vi "SwissSPAD Live_Settings Storage.vi"(6 "Set/Get(F)":bool, 7 "Settings List":T15=enum."FPGA:Bottom Bitfile Path", 8 "Error In":errorcluster, 11 "Variant Data in":variant) -> (0 "Error Out":errorcluster, 3 "Variant Data out":variant)   [LabVIEW 2021]
uses:
  SwissSPAD Live_Settings List.ctl
  SwissSPAD Live_SS2 DAQ Parameters 3.ctl
  SwissSPAD Live_SS2 Gate Definition.ctl
  SwissSPAD Live_File Information.ctl
  SwissSPAD Live_SS2 Gate Configuration.ctl
  SwissSPAD Live_Image ROI Information.ctl
  Phasor/Image Binning Options.ctl
  SwissSPAD Live_SS3 DAQ Parameters.ctl
  SwissSPAD Live_SS3 Gate Definition.ctl
  SS3 Gate Width Definition Mode.ctl
  SwissSPAD Live_SS3 Displayed Image v2.ctl
  SwissSPAD Live_SSx PCB Version.ctl
  SwissSPAD Live_Image Display Options.ctl
  SwissSPAD Live_FPGA Data to Display.ctl
  281105eb-bd69-41f7-a288-d5f8cce70846.vi
panel:
  in  "Tab Control":T1(tab)
  in  "Top Half":bool
  in  "Top FPGA Serial Number":string
  in  "Top Bitstream Version":string
  in  "Top Bitfile Path":path
  in  "Bottom Half":bool
  in  "Detector PCB Version":T2
  in  "Bottom FPGA Serial Number":string
  in  "Bottom Bitstream Version":string
  in  "Bottom BitFile Path":path
  in  "Auto Reset FPGA":bool
  in  "Microlens":bool
  in  "SS3 DAQ Parameters":T3={"10 bits"=FALSE, "# Exposure Sequences"=0, "# 1-bit Frame per Gate"=255, "Gate Shift"=0, "# Gate Pairs per Set"=0, "# Sets"=1, "Laser Period"=0.0, "Sync Period"=0.0, "Gate Offset"=0, "Auto-adjust Gate Offset"=FALSE, "Gate Definition"={"gs_psincdec_0"=0, "gs_psincdec_1"=0, "gs_no_shift_adj_1"=0, "gate_adj_2"=0}, "Gate Width (ns)"=0.0, "Reversed Shift"=FALSE, "Intensity Mode"=FALSE, "Gate Definition Mode"=enum."Item 0"} {"Gate Width (ns)" min=0.0 max=100.0 format="%#_5g"; "# Sets" min=1}
  in  "Buffer Size (# 8-bit Gates)":u32=1 min=1
  in  "SS2 DAQ Parameters":T6 {"Sync Period" min=0.0 max=4.294967295; "Laser Period" min=0.0 max=4.294967295}
  in  "Gate Configuration Definitions":T8[](array[typedef])
  in  "FPGA Data to Display":T9
  in  "Use Histogram Cursors":bool
  in  "Image Display Options":T10 {"Percentile" min=0 max=100}
  in  "Image Binning Options":T11={"Use Image Binning"=FALSE, "X Bin"=1, "Y Bin"=1} {"Y Bin" min=1; "X Bin" min=1}
  in  "Image ROI Information":T12
  in  "SS3 Displayed Image":T13
  in  "Save Sum of All Gates Preview":bool
  in  "SS3 Gate Slip Correction":bool
  in  "Delay between Datasets":dbl[unit]
  in  "Scrambled File Flag":bool
  in  "# Datasets in Series":i32=1 min=1
  in  "File Information":T14={"File Folder"=path "", "File Name"="", "File Index"=0, "Author"="", "Sample"="", "Compression"=FALSE, "Compression Level"=9} {"Compression Level" max=9}
  in  "SS3 Hot Pixel Mismatch Detection":bool
  in  "Histogram Bin Size":i32=256 min=1 step=1
  in  "Verbose Saving":bool
  in  "Verbose Settings":bool
  in  "Use Image Display Options":bool
  in  "# Histogram Bins":i32=1 min=1 step=1
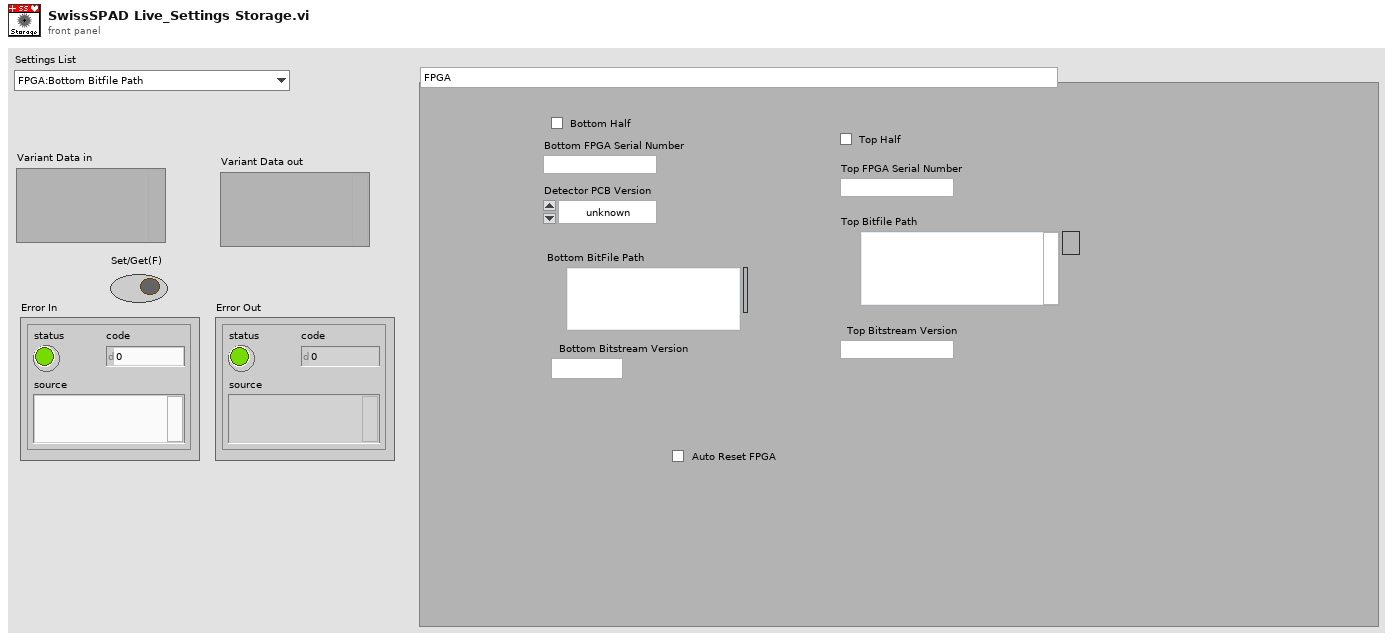
[diagram p1: front panel]
types:
  T1 = enum32{"FPGA", "Acquisition Parameters", "Image Parameters", "File Information", "UI Settings"}
  T2 = typedef "SwissSPAD Live_SSx PCB Version.ctl" = enum16{"unknown", "SS2 PCB1", "SS2 PCB2", "SS3 PCB1"}
  T3 = typedef "SwissSPAD Live_SS3 DAQ Parameters.ctl" = cluster{"10 bits":bool, "# Exposure Sequences":u32, "# 1-bit Frame per Gate":u32, "Gate Shift":u32, "# Gate Pairs per Set":u32, "# Sets":u32, "Laser Period":dbl[unit], "Sync Period":dbl[unit], "Gate Offset":u32, "Auto-adjust Gate Offset":bool, "Gate Definition":T4, "Gate Width (ns)":dbl, "Reversed Shift":bool, "Intensity Mode":bool, "Gate Definition Mode":T5}
  T4 = typedef "SwissSPAD Live_SS3 Gate Definition.ctl" = cluster{"gs_psincdec_0":u32, "gs_psincdec_1":u32, "gs_no_shift_adj_1":u32, "gate_adj_2":u32}
  T5 = typedef "SS3 Gate Width Definition Mode.ctl" = enum32{"Item 0", "Item 1"}
  T6 = typedef "SwissSPAD Live_SS2 DAQ Parameters 3.ctl" = cluster{"10 bits":bool, "# Exposure Sequences":u32, "# 1-bit Frame per Gate":u32, "Gate Shift":u32, "# Gates per Set":u32, "# Sets":u32, "Laser Period":dbl[unit], "Sync Period":dbl[unit], "Gate Offset":u32, "Auto-adjust Gate Offset":bool, "Gate Definition":T7, "Reversed Shift":bool}
  T7 = typedef "SwissSPAD Live_SS2 Gate Definition.ctl" = cluster{"gs_psincdec_0":u32, "gs_psincdec_1":u32, "gs_psincdec_2":u32, "gs_psincdec_3":u32, "gs_no_shift_adj_1":u32, "gs_no_shift_adj_2":u32, "gs_no_shift_adj_3":u32}
  T8 = typedef "SwissSPAD Live_SS2 Gate Configuration.ctl" = cluster{"Gate Configuration":string, "Gate Offset":u32, "Gate Definition":T7}
  T9 = typedef "SwissSPAD Live_FPGA Data to Display.ctl" = enum16{"Bottom FPGA", "Top FPGA", "Both"}
  T10 = typedef "SwissSPAD Live_Image Display Options.ctl" = cluster{"Remove Screamers":bool, "Delta":sgl, "Equalize Histogram":bool, "Percentile":sgl, "Hot Pixel Mask Image":path, "Use Hot Pixel Mask":bool}
  T11 = typedef "Image Binning Options.ctl" = cluster{"Use Image Binning":bool, "X Bin":i32, "Y Bin":i32}
  T12 = typedef "SwissSPAD Live_Image ROI Information.ctl" = cluster{"Save ROI Only":bool, "Left":u16, "Top":u16, "Right":u16, "Bottom":u16, "Use Current ROI":bool}
  T13 = typedef "SwissSPAD Live_SS3 Displayed Image v2.ctl" = enum16{"G2 Gate", "INT Gate", "INT - G2"}
  T14 = typedef "SwissSPAD Live_File Information.ctl" = cluster{"File Folder":path, "File Name":string, "File Index":u32, "Author":string, "Sample":string, "Compression":bool, "Compression Level":u8}
  T15 = typedef "SwissSPAD Live_Settings List.ctl" = enum16{"FPGA:Bottom Half", "FPGA:Top Half", "FPGA:Bottom Bitfile Path", "FPGA:Top Bitfile Path", "FPGA:Bottom Bitstream Version", "FPGA:Top Bitstream Version", "FPGA:Auto Reset FPGA", "FPGA:Bottom FPGA Serial Number", "FPGA:Top FPGA Serial Number", "FPGA:Detector PCB Version", "Acquisition Parameters:Microlens", "Acquisition Parameters:SS2 DAQ Parameters", "Acquisition Parameters:Gate Configuration Array", "Acquisition Parameters:SS3 DAQ Parameters", "Acquisition Parameters:Buffer Size (# 8-bit Gates)", "File Information:File Information", "File Information:# Datasets in Series", "File Information:Scrambled File Flag", "File Information:SS3 Gate Slip Correction", "File Information:SS3 Hot Pixel Mismatch Detection", "File Information:Delay between Datasets", "File Information:Save Sum of All Gates Preview", "Image Parameters:Image ROI Information", "Image Parameters:Image Binning Options", "Image Parameters:SS3 Displayed Image", "Image Parameters:Image Display Options", "Image Parameters:Use Histogram Cursors", "Image Parameter:FPGA Data to Display", "UI Settings:Histogram Bins Number", "UI Settings:Histogram Bin Size", "UI Settings:Use Image Display Options", "UI Settings:Verbose Settings", "UI Settings:Verbose Saving"}
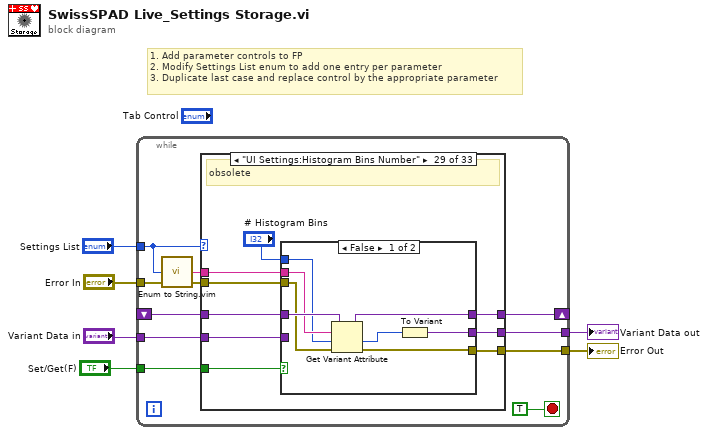
[diagram p0: block diagram]
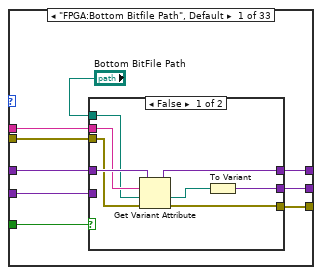
[diagram p2: hidden frame]
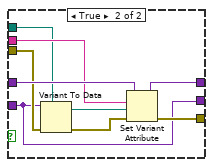
[diagram p3: hidden frame]
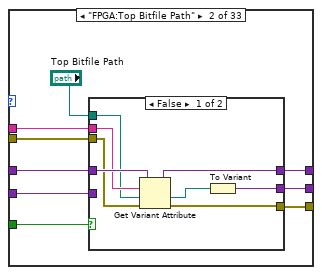
[diagram p4: hidden frame]
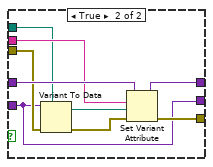
[diagram p5: hidden frame]
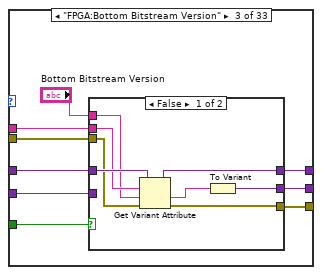
[diagram p6: hidden frame]
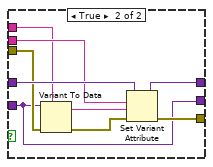
[diagram p7: hidden frame]
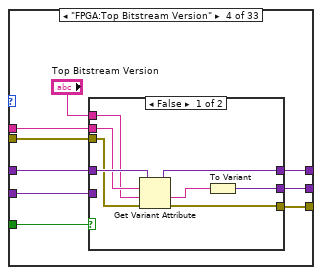
[diagram p8: hidden frame]
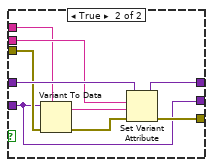
[diagram p9: hidden frame]
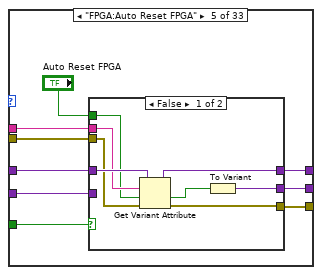
[diagram p10: hidden frame]
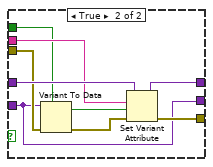
[diagram p11: hidden frame]
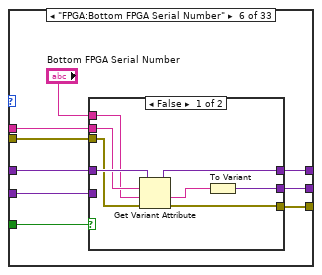
[diagram p12: hidden frame]
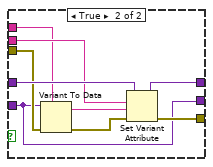
[diagram p13: hidden frame]
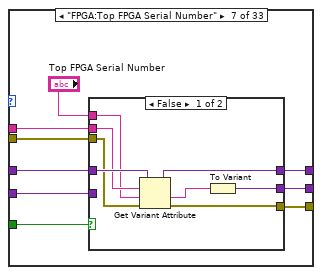
[diagram p14: hidden frame]
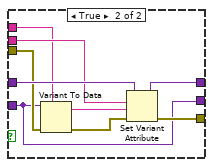
[diagram p15: hidden frame]
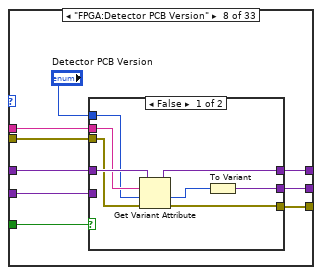
[diagram p16: hidden frame]
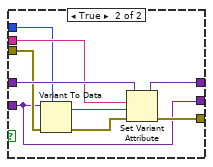
[diagram p17: hidden frame]
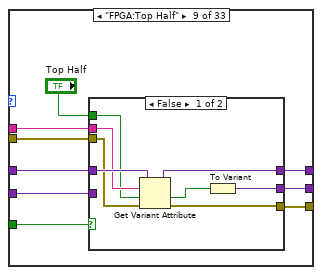
[diagram p18: hidden frame]
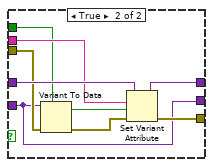
[diagram p19: hidden frame]
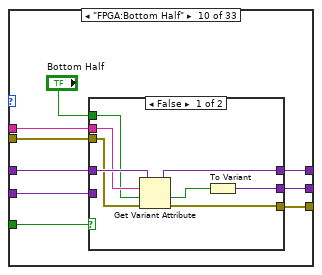
[diagram p20: hidden frame]
diagram:
  # "1. Add parameter controls to FP\n2. Modify Settings List enum to add one entry per parameter\n3. Duplicate last case and replace control by the appropriate parameter"
  n1 = while {
    tunnel: "Settings List" -> [w9]
    tunnel: "Error In" -> [w7]
    tunnel: "Set/Get(F)" -> [w15]
    shift-right: [w13] -> _
    shift-left: _ -> [w14]
    tunnel: "Variant Data in" -> [w12]
    tunnel: [w11] -> w2
    tunnel: [w10] -> w1
    stop <- TRUE stop-if-true
    n2 = call "Enum to String.vim"("Enum"=w9) -> ("String"=w8:string)
    n3 = case shown="\"UI Settings:Histogram Bins Number\"" w9 {
      tunnel: w15 -> [w25 w51 w77 w103 w129 w155 w181 w207 w233 w259 w285 w311 w337 w363 w389 w415 w441 w467 w493 w519 w545 w571 w597 w623 w649 w675 w701 w727 w753 w779 w805 w831 w857]
      tunnel: w14 -> [w24 w50 w76 w102 w128 w154 w180 w206 w232 w258 w284 w310 w336 w362 w388 w414 w440 w466 w492 w518 w544 w570 w596 w622 w648 w674 w700 w726 w752 w778 w804 w830 w856]
      tunnel: w8 -> [w23 w49 w75 w101 w127 w153 w179 w205 w231 w257 w283 w309 w335 w361 w387 w413 w439 w465 w491 w517 w543 w569 w595 w621 w647 w673 w699 w725 w751 w777 w803 w829 w855]
      tunnel: [w22 w48 w74 w100 w126 w152 w178 w204 w230 w256 w282 w308 w334 w360 w386 w412 w438 w464 w490 w516 w542 w568 w594 w620 w646 w672 w698 w724 w750 w776 w802 w828 w854] -> w13
      tunnel: w7 -> [w21 w47 w73 w99 w125 w151 w177 w203 w229 w255 w281 w307 w333 w359 w385 w411 w437 w463 w489 w515 w541 w567 w593 w619 w645 w671 w697 w723 w749 w775 w801 w827 w853]
      tunnel: w12 -> [w20 w46 w72 w98 w124 w150 w176 w202 w228 w254 w280 w306 w332 w358 w384 w410 w436 w462 w488 w514 w540 w566 w592 w618 w644 w670 w696 w722 w748 w774 w800 w826 w852]
      tunnel: [w19 w45 w71 w97 w123 w149 w175 w201 w227 w253 w279 w305 w331 w357 w383 w409 w435 w461 w487 w513 w539 w565 w591 w617 w643 w669 w695 w721 w747 w773 w799 w825 w851] -> w11
      tunnel: [w18 w44 w70 w96 w122 w148 w174 w200 w226 w252 w278 w304 w330 w356 w382 w408 w434 w460 w486 w512 w538 w564 w590 w616 w642 w668 w694 w720 w746 w772 w798 w824 w850] -> w10
      frame "FPGA:Bottom Bitfile Path", Default {
        n4 = case shown="False" w25 {
          tunnel: w24 -> [w33 w42]
          tunnel: w23 -> [w32 w41]
          tunnel: [w30 w40] -> w22
          tunnel: "Bottom BitFile Path" -> [w27 w39]
          tunnel: w21 -> [w31 w38]
          tunnel: w20 -> [_ w34]
          tunnel: [w29 w35] -> w19
          tunnel: [w26 w34] -> w18
          frame False {
            n5 = Get Variant Attribute(Variant=w33, name=w32, default value (empty Variant)=w27, error in=w31) -> (duplicate Variant=w30:variant, value=w28:path, error out=w29:errorcluster)  [unwired: 1 out]
            n6 = To Variant(anything=w28) -> (Variant=w26:variant)
          }
          frame True {
            n7 = Variant To Data(error in=w38, type=w39, Variant=w34) -> (data=w37:path, error out=w36:errorcluster)
            n8 = Set Variant Attribute(Variant=w42, name=w41, value=w37, error in=w36) -> (Variant out=w40:variant, error out=w35:errorcluster)  [unwired: 1 out]
          }
        }
      }
      frame "FPGA:Top Bitfile Path" {
        n9 = case shown="False" w51 {
          tunnel: w50 -> [w59 w68]
          tunnel: w49 -> [w58 w67]
          tunnel: [w56 w66] -> w48
          tunnel: "Top Bitfile Path" -> [w53 w65]
          tunnel: w47 -> [w57 w64]
          tunnel: w46 -> [_ w60]
          tunnel: [w55 w61] -> w45
          tunnel: [w52 w60] -> w44
          frame False {
            n10 = Get Variant Attribute(Variant=w59, name=w58, default value (empty Variant)=w53, error in=w57) -> (duplicate Variant=w56:variant, value=w54:path, error out=w55:errorcluster)  [unwired: 1 out]
            n11 = To Variant(anything=w54) -> (Variant=w52:variant)
          }
          frame True {
            n12 = Variant To Data(error in=w64, type=w65, Variant=w60) -> (data=w63:path, error out=w62:errorcluster)
            n13 = Set Variant Attribute(Variant=w68, name=w67, value=w63, error in=w62) -> (Variant out=w66:variant, error out=w61:errorcluster)  [unwired: 1 out]
          }
        }
      }
      frame "FPGA:Bottom Bitstream Version" {
        n14 = case shown="False" w77 {
          tunnel: w76 -> [w85 w94]
          tunnel: w75 -> [w84 w93]
          tunnel: [w82 w92] -> w74
          tunnel: "Bottom Bitstream Version" -> [w79 w91]
          tunnel: w73 -> [w83 w90]
          tunnel: w72 -> [_ w86]
          tunnel: [w81 w87] -> w71
          tunnel: [w78 w86] -> w70
          frame False {
            n15 = Get Variant Attribute(Variant=w85, name=w84, default value (empty Variant)=w79, error in=w83) -> (duplicate Variant=w82:variant, value=w80:string, error out=w81:errorcluster)  [unwired: 1 out]
            n16 = To Variant(anything=w80) -> (Variant=w78:variant)
          }
          frame True {
            n17 = Variant To Data(error in=w90, type=w91, Variant=w86) -> (data=w89:string, error out=w88:errorcluster)
            n18 = Set Variant Attribute(Variant=w94, name=w93, value=w89, error in=w88) -> (Variant out=w92:variant, error out=w87:errorcluster)  [unwired: 1 out]
          }
        }
      }
      frame "FPGA:Top Bitstream Version" {
        n19 = case shown="False" w103 {
          tunnel: w102 -> [w111 w120]
          tunnel: w101 -> [w110 w119]
          tunnel: [w108 w118] -> w100
          tunnel: "Top Bitstream Version" -> [w105 w117]
          tunnel: w99 -> [w109 w116]
          tunnel: w98 -> [_ w112]
          tunnel: [w107 w113] -> w97
          tunnel: [w104 w112] -> w96
          frame False {
            n20 = Get Variant Attribute(Variant=w111, name=w110, default value (empty Variant)=w105, error in=w109) -> (duplicate Variant=w108:variant, value=w106:string, error out=w107:errorcluster)  [unwired: 1 out]
            n21 = To Variant(anything=w106) -> (Variant=w104:variant)
          }
          frame True {
            n22 = Variant To Data(error in=w116, type=w117, Variant=w112) -> (data=w115:string, error out=w114:errorcluster)
            n23 = Set Variant Attribute(Variant=w120, name=w119, value=w115, error in=w114) -> (Variant out=w118:variant, error out=w113:errorcluster)  [unwired: 1 out]
          }
        }
      }
      frame "FPGA:Auto Reset FPGA" {
        n24 = case shown="False" w129 {
          tunnel: w128 -> [w137 w146]
          tunnel: w127 -> [w136 w145]
          tunnel: [w134 w144] -> w126
          tunnel: "Auto Reset FPGA" -> [w131 w143]
          tunnel: w125 -> [w135 w142]
          tunnel: w124 -> [_ w138]
          tunnel: [w133 w139] -> w123
          tunnel: [w130 w138] -> w122
          frame False {
            n25 = Get Variant Attribute(Variant=w137, name=w136, default value (empty Variant)=w131, error in=w135) -> (duplicate Variant=w134:variant, value=w132:bool, error out=w133:errorcluster)  [unwired: 1 out]
            n26 = To Variant(anything=w132) -> (Variant=w130:variant)
          }
          frame True {
            n27 = Variant To Data(error in=w142, type=w143, Variant=w138) -> (data=w141:bool, error out=w140:errorcluster)
            n28 = Set Variant Attribute(Variant=w146, name=w145, value=w141, error in=w140) -> (Variant out=w144:variant, error out=w139:errorcluster)  [unwired: 1 out]
          }
        }
      }
      frame "FPGA:Bottom FPGA Serial Number" {
        n29 = case shown="False" w155 {
          tunnel: w154 -> [w163 w172]
          tunnel: w153 -> [w162 w171]
          tunnel: [w160 w170] -> w152
          tunnel: "Bottom FPGA Serial Number" -> [w157 w169]
          tunnel: w151 -> [w161 w168]
          tunnel: w150 -> [_ w164]
          tunnel: [w159 w165] -> w149
          tunnel: [w156 w164] -> w148
          frame False {
            n30 = Get Variant Attribute(Variant=w163, name=w162, default value (empty Variant)=w157, error in=w161) -> (duplicate Variant=w160:variant, value=w158:string, error out=w159:errorcluster)  [unwired: 1 out]
            n31 = To Variant(anything=w158) -> (Variant=w156:variant)
          }
          frame True {
            n32 = Variant To Data(error in=w168, type=w169, Variant=w164) -> (data=w167:string, error out=w166:errorcluster)
            n33 = Set Variant Attribute(Variant=w172, name=w171, value=w167, error in=w166) -> (Variant out=w170:variant, error out=w165:errorcluster)  [unwired: 1 out]
          }
        }
      }
      frame "FPGA:Top FPGA Serial Number" {
        n34 = case shown="False" w181 {
          tunnel: w180 -> [w189 w198]
          tunnel: w179 -> [w188 w197]
          tunnel: [w186 w196] -> w178
          tunnel: "Top FPGA Serial Number" -> [w183 w195]
          tunnel: w177 -> [w187 w194]
          tunnel: w176 -> [_ w190]
          tunnel: [w185 w191] -> w175
          tunnel: [w182 w190] -> w174
          frame False {
            n35 = Get Variant Attribute(Variant=w189, name=w188, default value (empty Variant)=w183, error in=w187) -> (duplicate Variant=w186:variant, value=w184:string, error out=w185:errorcluster)  [unwired: 1 out]
            n36 = To Variant(anything=w184) -> (Variant=w182:variant)
          }
          frame True {
            n37 = Variant To Data(error in=w194, type=w195, Variant=w190) -> (data=w193:string, error out=w192:errorcluster)
            n38 = Set Variant Attribute(Variant=w198, name=w197, value=w193, error in=w192) -> (Variant out=w196:variant, error out=w191:errorcluster)  [unwired: 1 out]
          }
        }
      }
      frame "FPGA:Detector PCB Version" {
        n39 = case shown="False" w207 {
          tunnel: w206 -> [w215 w224]
          tunnel: w205 -> [w214 w223]
          tunnel: [w212 w222] -> w204
          tunnel: "Detector PCB Version" -> [w209 w221]
          tunnel: w203 -> [w213 w220]
          tunnel: w202 -> [_ w216]
          tunnel: [w211 w217] -> w201
          tunnel: [w208 w216] -> w200
          frame False {
            n40 = Get Variant Attribute(Variant=w215, name=w214, default value (empty Variant)=w209, error in=w213) -> (duplicate Variant=w212:variant, value=w210:T2, error out=w211:errorcluster)  [unwired: 1 out]
            n41 = To Variant(anything=w210) -> (Variant=w208:variant)
          }
          frame True {
            n42 = Variant To Data(error in=w220, type=w221, Variant=w216) -> (data=w219:T2, error out=w218:errorcluster)
            n43 = Set Variant Attribute(Variant=w224, name=w223, value=w219, error in=w218) -> (Variant out=w222:variant, error out=w217:errorcluster)  [unwired: 1 out]
          }
        }
      }
      frame "FPGA:Top Half" {
        n44 = case shown="False" w233 {
          tunnel: w232 -> [w241 w250]
          tunnel: w231 -> [w240 w249]
          tunnel: [w238 w248] -> w230
          tunnel: "Top Half" -> [w235 w247]
          tunnel: w229 -> [w239 w246]
          tunnel: w228 -> [_ w242]
          tunnel: [w237 w243] -> w227
          tunnel: [w234 w242] -> w226
          frame False {
            n45 = Get Variant Attribute(Variant=w241, name=w240, default value (empty Variant)=w235, error in=w239) -> (duplicate Variant=w238:variant, value=w236:bool, error out=w237:errorcluster)  [unwired: 1 out]
            n46 = To Variant(anything=w236) -> (Variant=w234:variant)
          }
          frame True {
            n47 = Variant To Data(error in=w246, type=w247, Variant=w242) -> (data=w245:bool, error out=w244:errorcluster)
            n48 = Set Variant Attribute(Variant=w250, name=w249, value=w245, error in=w244) -> (Variant out=w248:variant, error out=w243:errorcluster)  [unwired: 1 out]
          }
        }
      }
      frame "FPGA:Bottom Half" {
        n49 = case shown="False" w259 {
          tunnel: w258 -> [w267 w276]
          tunnel: w257 -> [w266 w275]
          tunnel: [w264 w274] -> w256
          tunnel: "Bottom Half" -> [w261 w273]
          tunnel: w255 -> [w265 w272]
          tunnel: w254 -> [_ w268]
          tunnel: [w263 w269] -> w253
          tunnel: [w260 w268] -> w252
          frame False {
            n50 = Get Variant Attribute(Variant=w267, name=w266, default value (empty Variant)=w261, error in=w265) -> (duplicate Variant=w264:variant, value=w262:bool, error out=w263:errorcluster)  [unwired: 1 out]
            n51 = To Variant(anything=w262) -> (Variant=w260:variant)
          }
          frame True {
            n52 = Variant To Data(error in=w272, type=w273, Variant=w268) -> (data=w271:bool, error out=w270:errorcluster)
            n53 = Set Variant Attribute(Variant=w276, name=w275, value=w271, error in=w270) -> (Variant out=w274:variant, error out=w269:errorcluster)  [unwired: 1 out]
          }
        }
      }
      frame "Acquisition Parameters:Microlens" {
        n54 = case shown="False" w285 {
          tunnel: w284 -> [w293 w302]
          tunnel: w283 -> [w292 w301]
          tunnel: [w290 w300] -> w282
          tunnel: "Microlens" -> [w287 w299]
          tunnel: w281 -> [w291 w298]
          tunnel: w280 -> [_ w294]
          tunnel: [w289 w295] -> w279
          tunnel: [w286 w294] -> w278
          frame False {
            n55 = Get Variant Attribute(Variant=w293, name=w292, default value (empty Variant)=w287, error in=w291) -> (duplicate Variant=w290:variant, value=w288:bool, error out=w289:errorcluster)  [unwired: 1 out]
            n56 = To Variant(anything=w288) -> (Variant=w286:variant)
          }
          frame True {
            n57 = Variant To Data(error in=w298, type=w299, Variant=w294) -> (data=w297:bool, error out=w296:errorcluster)
            n58 = Set Variant Attribute(Variant=w302, name=w301, value=w297, error in=w296) -> (Variant out=w300:variant, error out=w295:errorcluster)  [unwired: 1 out]
          }
        }
      }
      frame "Acquisition Parameters:SS2 DAQ Parameters" {
        n59 = case shown="False" w311 {
          tunnel: w310 -> [w319 w328]
          tunnel: w309 -> [w318 w327]
          tunnel: [w316 w326] -> w308
          tunnel: "SS2 DAQ Parameters" -> [w313 w325]
          tunnel: w307 -> [w317 w324]
          tunnel: w306 -> [_ w320]
          tunnel: [w315 w321] -> w305
          tunnel: [w312 w320] -> w304
          frame False {
            n60 = Get Variant Attribute(Variant=w319, name=w318, default value (empty Variant)=w313, error in=w317) -> (duplicate Variant=w316:variant, value=w314:T6, error out=w315:errorcluster)  [unwired: 1 out]
            n61 = To Variant(anything=w314) -> (Variant=w312:variant)
          }
          frame True {
            n62 = Variant To Data(error in=w324, type=w325, Variant=w320) -> (data=w323:T6, error out=w322:errorcluster)
            n63 = Set Variant Attribute(Variant=w328, name=w327, value=w323, error in=w322) -> (Variant out=w326:variant, error out=w321:errorcluster)  [unwired: 1 out]
          }
        }
      }
      frame "Acquisition Parameters:SS3 DAQ Parameters" {
        n64 = case shown="False" w337 {
          tunnel: w336 -> [w345 w354]
          tunnel: w335 -> [w344 w353]
          tunnel: [w342 w352] -> w334
          tunnel: "SS3 DAQ Parameters" -> [w339 w351]
          tunnel: w333 -> [w343 w350]
          tunnel: w332 -> [_ w346]
          tunnel: [w341 w347] -> w331
          tunnel: [w338 w346] -> w330
          frame False {
            n65 = Get Variant Attribute(Variant=w345, name=w344, default value (empty Variant)=w339, error in=w343) -> (duplicate Variant=w342:variant, value=w340:T3, error out=w341:errorcluster)  [unwired: 1 out]
            n66 = To Variant(anything=w340) -> (Variant=w338:variant)
          }
          frame True {
            n67 = Variant To Data(error in=w350, type=w351, Variant=w346) -> (data=w349:T3, error out=w348:errorcluster)
            n68 = Set Variant Attribute(Variant=w354, name=w353, value=w349, error in=w348) -> (Variant out=w352:variant, error out=w347:errorcluster)  [unwired: 1 out]
          }
        }
      }
      frame "Acquisition Parameters:Gate Configuration Array" {
        n69 = case shown="False" w363 {
          tunnel: w362 -> [w371 w380]
          tunnel: w361 -> [w370 w379]
          tunnel: [w368 w378] -> w360
          tunnel: "Gate Configuration Definitions" -> [w365 w377]
          tunnel: w359 -> [w369 w376]
          tunnel: w358 -> [_ w372]
          tunnel: [w367 w373] -> w357
          tunnel: [w364 w372] -> w356
          frame False {
            n70 = Get Variant Attribute(Variant=w371, name=w370, default value (empty Variant)=w365, error in=w369) -> (duplicate Variant=w368:variant, value=w366:T8[], error out=w367:errorcluster)  [unwired: 1 out]
            n71 = To Variant(anything=w366) -> (Variant=w364:variant)
          }
          frame True {
            n72 = Variant To Data(error in=w376, type=w377, Variant=w372) -> (data=w375:T8[], error out=w374:errorcluster)
            n73 = Set Variant Attribute(Variant=w380, name=w379, value=w375, error in=w374) -> (Variant out=w378:variant, error out=w373:errorcluster)  [unwired: 1 out]
          }
        }
      }
      frame "Acquisition Parameters:Buffer Size (# 8-bit Gates)" {
        n74 = case shown="False" w389 {
          tunnel: w388 -> [w397 w406]
          tunnel: w387 -> [w396 w405]
          tunnel: [w394 w404] -> w386
          tunnel: "Buffer Size (# 8-bit Gates)" -> [w391 w403]
          tunnel: w385 -> [w395 w402]
          tunnel: w384 -> [_ w398]
          tunnel: [w393 w399] -> w383
          tunnel: [w390 w398] -> w382
          frame False {
            n75 = Get Variant Attribute(Variant=w397, name=w396, default value (empty Variant)=w391, error in=w395) -> (duplicate Variant=w394:variant, value=w392:u32, error out=w393:errorcluster)  [unwired: 1 out]
            n76 = To Variant(anything=w392) -> (Variant=w390:variant)
          }
          frame True {
            n77 = Variant To Data(error in=w402, type=w403, Variant=w398) -> (data=w401:u32, error out=w400:errorcluster)
            n78 = Set Variant Attribute(Variant=w406, name=w405, value=w401, error in=w400) -> (Variant out=w404:variant, error out=w399:errorcluster)  [unwired: 1 out]
          }
        }
      }
      frame "File Information:File Information" {
        n79 = case shown="False" w415 {
          tunnel: w414 -> [w423 w432]
          tunnel: w413 -> [w422 w431]
          tunnel: [w420 w430] -> w412
          tunnel: "File Information" -> [w417 w429]
          tunnel: w411 -> [w421 w428]
          tunnel: w410 -> [_ w424]
          tunnel: [w419 w425] -> w409
          tunnel: [w416 w424] -> w408
          frame False {
            n80 = Get Variant Attribute(Variant=w423, name=w422, default value (empty Variant)=w417, error in=w421) -> (duplicate Variant=w420:variant, value=w418:T14, error out=w419:errorcluster)  [unwired: 1 out]
            n81 = To Variant(anything=w418) -> (Variant=w416:variant)
          }
          frame True {
            n82 = Variant To Data(error in=w428, type=w429, Variant=w424) -> (data=w427:T14, error out=w426:errorcluster)
            n83 = Set Variant Attribute(Variant=w432, name=w431, value=w427, error in=w426) -> (Variant out=w430:variant, error out=w425:errorcluster)  [unwired: 1 out]
          }
        }
      }
      frame "File Information:# Datasets in Series" {
        n84 = case shown="False" w441 {
          tunnel: w440 -> [w449 w458]
          tunnel: w439 -> [w448 w457]
          tunnel: [w446 w456] -> w438
          tunnel: "# Datasets in Series" -> [w443 w455]
          tunnel: w437 -> [w447 w454]
          tunnel: w436 -> [_ w450]
          tunnel: [w445 w451] -> w435
          tunnel: [w442 w450] -> w434
          frame False {
            n85 = Get Variant Attribute(Variant=w449, name=w448, default value (empty Variant)=w443, error in=w447) -> (duplicate Variant=w446:variant, value=w444:i32, error out=w445:errorcluster)  [unwired: 1 out]
            n86 = To Variant(anything=w444) -> (Variant=w442:variant)
          }
          frame True {
            n87 = Variant To Data(error in=w454, type=w455, Variant=w450) -> (data=w453:i32, error out=w452:errorcluster)
            n88 = Set Variant Attribute(Variant=w458, name=w457, value=w453, error in=w452) -> (Variant out=w456:variant, error out=w451:errorcluster)  [unwired: 1 out]
          }
        }
      }
      frame "File Information:Scrambled File Flag" {
        n89 = case shown="False" w467 {
          tunnel: w466 -> [w475 w484]
          tunnel: w465 -> [w474 w483]
          tunnel: [w472 w482] -> w464
          tunnel: "Scrambled File Flag" -> [w469 w481]
          tunnel: w463 -> [w473 w480]
          tunnel: w462 -> [_ w476]
          tunnel: [w471 w477] -> w461
          tunnel: [w468 w476] -> w460
          frame False {
            n90 = Get Variant Attribute(Variant=w475, name=w474, default value (empty Variant)=w469, error in=w473) -> (duplicate Variant=w472:variant, value=w470:bool, error out=w471:errorcluster)  [unwired: 1 out]
            n91 = To Variant(anything=w470) -> (Variant=w468:variant)
          }
          frame True {
            n92 = Variant To Data(error in=w480, type=w481, Variant=w476) -> (data=w479:bool, error out=w478:errorcluster)
            n93 = Set Variant Attribute(Variant=w484, name=w483, value=w479, error in=w478) -> (Variant out=w482:variant, error out=w477:errorcluster)  [unwired: 1 out]
          }
        }
      }
      frame "File Information:SS3 Gate Slip Correction" {
        n94 = case shown="False" w493 {
          tunnel: w492 -> [w501 w510]
          tunnel: w491 -> [w500 w509]
          tunnel: [w498 w508] -> w490
          tunnel: "SS3 Gate Slip Correction" -> [w495 w507]
          tunnel: w489 -> [w499 w506]
          tunnel: w488 -> [_ w502]
          tunnel: [w497 w503] -> w487
          tunnel: [w494 w502] -> w486
          frame False {
            n95 = Get Variant Attribute(Variant=w501, name=w500, default value (empty Variant)=w495, error in=w499) -> (duplicate Variant=w498:variant, value=w496:bool, error out=w497:errorcluster)  [unwired: 1 out]
            n96 = To Variant(anything=w496) -> (Variant=w494:variant)
          }
          frame True {
            n97 = Variant To Data(error in=w506, type=w507, Variant=w502) -> (data=w505:bool, error out=w504:errorcluster)
            n98 = Set Variant Attribute(Variant=w510, name=w509, value=w505, error in=w504) -> (Variant out=w508:variant, error out=w503:errorcluster)  [unwired: 1 out]
          }
        }
      }
      frame "File Information:SS3 Hot Pixel Mismatch Detection" {
        n99 = case shown="False" w519 {
          tunnel: w518 -> [w527 w536]
          tunnel: w517 -> [w526 w535]
          tunnel: [w524 w534] -> w516
          tunnel: "SS3 Hot Pixel Mismatch Detection" -> [w521 w533]
          tunnel: w515 -> [w525 w532]
          tunnel: w514 -> [_ w528]
          tunnel: [w523 w529] -> w513
          tunnel: [w520 w528] -> w512
          frame False {
            n100 = Get Variant Attribute(Variant=w527, name=w526, default value (empty Variant)=w521, error in=w525) -> (duplicate Variant=w524:variant, value=w522:bool, error out=w523:errorcluster)  [unwired: 1 out]
            n101 = To Variant(anything=w522) -> (Variant=w520:variant)
          }
          frame True {
            n102 = Variant To Data(error in=w532, type=w533, Variant=w528) -> (data=w531:bool, error out=w530:errorcluster)
            n103 = Set Variant Attribute(Variant=w536, name=w535, value=w531, error in=w530) -> (Variant out=w534:variant, error out=w529:errorcluster)  [unwired: 1 out]
          }
        }
      }
      frame "File Information:Save Sum of All Gates Preview" {
        n104 = case shown="False" w545 {
          tunnel: w544 -> [w553 w562]
          tunnel: w543 -> [w552 w561]
          tunnel: [w550 w560] -> w542
          tunnel: "Save Sum of All Gates Preview" -> [w547 w559]
          tunnel: w541 -> [w551 w558]
          tunnel: w540 -> [_ w554]
          tunnel: [w549 w555] -> w539
          tunnel: [w546 w554] -> w538
          frame False {
            n105 = Get Variant Attribute(Variant=w553, name=w552, default value (empty Variant)=w547, error in=w551) -> (duplicate Variant=w550:variant, value=w548:bool, error out=w549:errorcluster)  [unwired: 1 out]
            n106 = To Variant(anything=w548) -> (Variant=w546:variant)
          }
          frame True {
            n107 = Variant To Data(error in=w558, type=w559, Variant=w554) -> (data=w557:bool, error out=w556:errorcluster)
            n108 = Set Variant Attribute(Variant=w562, name=w561, value=w557, error in=w556) -> (Variant out=w560:variant, error out=w555:errorcluster)  [unwired: 1 out]
          }
        }
      }
      frame "File Information:Delay between Datasets" {
        n109 = case shown="False" w571 {
          tunnel: w570 -> [w579 w588]
          tunnel: w569 -> [w578 w587]
          tunnel: [w576 w586] -> w568
          tunnel: "Delay between Datasets" -> [w573 w585]
          tunnel: w567 -> [w577 w584]
          tunnel: w566 -> [_ w580]
          tunnel: [w575 w581] -> w565
          tunnel: [w572 w580] -> w564
          frame False {
            n110 = Get Variant Attribute(Variant=w579, name=w578, default value (empty Variant)=w573, error in=w577) -> (duplicate Variant=w576:variant, value=w574:dbl[unit], error out=w575:errorcluster)  [unwired: 1 out]
            n111 = To Variant(anything=w574) -> (Variant=w572:variant)
          }
          frame True {
            n112 = Variant To Data(error in=w584, type=w585, Variant=w580) -> (data=w583:dbl[unit], error out=w582:errorcluster)
            n113 = Set Variant Attribute(Variant=w588, name=w587, value=w583, error in=w582) -> (Variant out=w586:variant, error out=w581:errorcluster)  [unwired: 1 out]
          }
        }
      }
      frame "Image Parameters:Image ROI Information" {
        n114 = case shown="False" w597 {
          tunnel: w596 -> [w605 w614]
          tunnel: w595 -> [w604 w613]
          tunnel: [w602 w612] -> w594
          tunnel: "Image ROI Information" -> [w599 w611]
          tunnel: w593 -> [w603 w610]
          tunnel: w592 -> [_ w606]
          tunnel: [w601 w607] -> w591
          tunnel: [w598 w606] -> w590
          frame False {
            n115 = Get Variant Attribute(Variant=w605, name=w604, default value (empty Variant)=w599, error in=w603) -> (duplicate Variant=w602:variant, value=w600:T12, error out=w601:errorcluster)  [unwired: 1 out]
            n116 = To Variant(anything=w600) -> (Variant=w598:variant)
          }
          frame True {
            n117 = Variant To Data(error in=w610, type=w611, Variant=w606) -> (data=w609:T12, error out=w608:errorcluster)
            n118 = Set Variant Attribute(Variant=w614, name=w613, value=w609, error in=w608) -> (Variant out=w612:variant, error out=w607:errorcluster)  [unwired: 1 out]
          }
        }
      }
      frame "Image Parameters:Image Binning Options" {
        n119 = case shown="False" w623 {
          tunnel: w622 -> [w631 w640]
          tunnel: w621 -> [w630 w639]
          tunnel: [w628 w638] -> w620
          tunnel: "Image Binning Options" -> [w625 w637]
          tunnel: w619 -> [w629 w636]
          tunnel: w618 -> [_ w632]
          tunnel: [w627 w633] -> w617
          tunnel: [w624 w632] -> w616
          frame False {
            n120 = Get Variant Attribute(Variant=w631, name=w630, default value (empty Variant)=w625, error in=w629) -> (duplicate Variant=w628:variant, value=w626:T11, error out=w627:errorcluster)  [unwired: 1 out]
            n121 = To Variant(anything=w626) -> (Variant=w624:variant)
          }
          frame True {
            n122 = Variant To Data(error in=w636, type=w637, Variant=w632) -> (data=w635:T11, error out=w634:errorcluster)
            n123 = Set Variant Attribute(Variant=w640, name=w639, value=w635, error in=w634) -> (Variant out=w638:variant, error out=w633:errorcluster)  [unwired: 1 out]
          }
        }
      }
      frame "Image Parameters:SS3 Displayed Image" {
        n124 = case shown="False" w649 {
          tunnel: w648 -> [w657 w666]
          tunnel: w647 -> [w656 w665]
          tunnel: [w654 w664] -> w646
          tunnel: "SS3 Displayed Image" -> [w651 w663]
          tunnel: w645 -> [w655 w662]
          tunnel: w644 -> [_ w658]
          tunnel: [w653 w659] -> w643
          tunnel: [w650 w658] -> w642
          frame False {
            n125 = Get Variant Attribute(Variant=w657, name=w656, default value (empty Variant)=w651, error in=w655) -> (duplicate Variant=w654:variant, value=w652:T13, error out=w653:errorcluster)  [unwired: 1 out]
            n126 = To Variant(anything=w652) -> (Variant=w650:variant)
          }
          frame True {
            n127 = Variant To Data(error in=w662, type=w663, Variant=w658) -> (data=w661:T13, error out=w660:errorcluster)
            n128 = Set Variant Attribute(Variant=w666, name=w665, value=w661, error in=w660) -> (Variant out=w664:variant, error out=w659:errorcluster)  [unwired: 1 out]
          }
        }
      }
      frame "Image Parameters:Image Display Options" {
        n129 = case shown="False" w675 {
          tunnel: w674 -> [w683 w692]
          tunnel: w673 -> [w682 w691]
          tunnel: [w680 w690] -> w672
          tunnel: "Image Display Options" -> [w677 w689]
          tunnel: w671 -> [w681 w688]
          tunnel: w670 -> [_ w684]
          tunnel: [w679 w685] -> w669
          tunnel: [w676 w684] -> w668
          frame False {
            n130 = Get Variant Attribute(Variant=w683, name=w682, default value (empty Variant)=w677, error in=w681) -> (duplicate Variant=w680:variant, value=w678:T10, error out=w679:errorcluster)  [unwired: 1 out]
            n131 = To Variant(anything=w678) -> (Variant=w676:variant)
          }
          frame True {
            n132 = Variant To Data(error in=w688, type=w689, Variant=w684) -> (data=w687:T10, error out=w686:errorcluster)
            n133 = Set Variant Attribute(Variant=w692, name=w691, value=w687, error in=w686) -> (Variant out=w690:variant, error out=w685:errorcluster)  [unwired: 1 out]
          }
        }
      }
      frame "Image Parameters:Use Histogram Cursors" {
        n134 = case shown="True" w701 {
          tunnel: w700 -> [w709 w718]
          tunnel: w699 -> [w708 w717]
          tunnel: [w706 w716] -> w698
          tunnel: "Use Histogram Cursors" -> [w703 w715]
          tunnel: w697 -> [w707 w714]
          tunnel: w696 -> [_ w710]
          tunnel: [w705 w711] -> w695
          tunnel: [w702 w710] -> w694
          frame False {
            n135 = Get Variant Attribute(Variant=w709, name=w708, default value (empty Variant)=w703, error in=w707) -> (duplicate Variant=w706:variant, value=w704:bool, error out=w705:errorcluster)  [unwired: 1 out]
            n136 = To Variant(anything=w704) -> (Variant=w702:variant)
          }
          frame True {
            n137 = Variant To Data(error in=w714, type=w715, Variant=w710) -> (data=w713:bool, error out=w712:errorcluster)
            n138 = Set Variant Attribute(Variant=w718, name=w717, value=w713, error in=w712) -> (Variant out=w716:variant, error out=w711:errorcluster)  [unwired: 1 out]
          }
        }
      }
      frame "Image Parameter:FPGA Data to Display" {
        n139 = case shown="True" w727 {
          tunnel: w726 -> [w735 w744]
          tunnel: w725 -> [w734 w743]
          tunnel: [w732 w742] -> w724
          tunnel: "FPGA Data to Display" -> [w729 w741]
          tunnel: w723 -> [w733 w740]
          tunnel: w722 -> [_ w736]
          tunnel: [w731 w737] -> w721
          tunnel: [w728 w736] -> w720
          frame False {
            n140 = Get Variant Attribute(Variant=w735, name=w734, default value (empty Variant)=w729, error in=w733) -> (duplicate Variant=w732:variant, value=w730:T9, error out=w731:errorcluster)  [unwired: 1 out]
            n141 = To Variant(anything=w730) -> (Variant=w728:variant)
          }
          frame True {
            n142 = Variant To Data(error in=w740, type=w741, Variant=w736) -> (data=w739:T9, error out=w738:errorcluster)
            n143 = Set Variant Attribute(Variant=w744, name=w743, value=w739, error in=w738) -> (Variant out=w742:variant, error out=w737:errorcluster)  [unwired: 1 out]
          }
        }
      }
      frame "UI Settings:Histogram Bins Number" {
        # "obsolete"
        n144 = case shown="False" w753 {
          tunnel: w752 -> [w761 w770]
          tunnel: w751 -> [w760 w769]
          tunnel: [w758 w768] -> w750
          tunnel: "# Histogram Bins" -> [w755 w767]
          tunnel: w749 -> [w759 w766]
          tunnel: w748 -> [_ w762]
          tunnel: [w757 w763] -> w747
          tunnel: [w754 w762] -> w746
          frame False {
            n145 = Get Variant Attribute(Variant=w761, name=w760, default value (empty Variant)=w755, error in=w759) -> (duplicate Variant=w758:variant, value=w756:i32, error out=w757:errorcluster)  [unwired: 1 out]
            n146 = To Variant(anything=w756) -> (Variant=w754:variant)
          }
          frame True {
            n147 = Variant To Data(error in=w766, type=w767, Variant=w762) -> (data=w765:i32, error out=w764:errorcluster)
            n148 = Set Variant Attribute(Variant=w770, name=w769, value=w765, error in=w764) -> (Variant out=w768:variant, error out=w763:errorcluster)  [unwired: 1 out]
          }
        }
      }
      frame "UI Settings:Histogram Bin Size" {
        n149 = case shown="False" w779 {
          tunnel: w778 -> [w787 w796]
          tunnel: w777 -> [w786 w795]
          tunnel: [w784 w794] -> w776
          tunnel: "Histogram Bin Size" -> [w781 w793]
          tunnel: w775 -> [w785 w792]
          tunnel: w774 -> [_ w788]
          tunnel: [w783 w789] -> w773
          tunnel: [w780 w788] -> w772
          frame False {
            n150 = Get Variant Attribute(Variant=w787, name=w786, default value (empty Variant)=w781, error in=w785) -> (duplicate Variant=w784:variant, value=w782:i32, error out=w783:errorcluster)  [unwired: 1 out]
            n151 = To Variant(anything=w782) -> (Variant=w780:variant)
          }
          frame True {
            n152 = Variant To Data(error in=w792, type=w793, Variant=w788) -> (data=w791:i32, error out=w790:errorcluster)
            n153 = Set Variant Attribute(Variant=w796, name=w795, value=w791, error in=w790) -> (Variant out=w794:variant, error out=w789:errorcluster)  [unwired: 1 out]
          }
        }
      }
      frame "UI Settings:Use Image Display Options" {
        n154 = case shown="False" w805 {
          tunnel: w804 -> [w813 w822]
          tunnel: w803 -> [w812 w821]
          tunnel: [w810 w820] -> w802
          tunnel: "Use Image Display Options" -> [w807 w819]
          tunnel: w801 -> [w811 w818]
          tunnel: w800 -> [_ w814]
          tunnel: [w809 w815] -> w799
          tunnel: [w806 w814] -> w798
          frame False {
            n155 = Get Variant Attribute(Variant=w813, name=w812, default value (empty Variant)=w807, error in=w811) -> (duplicate Variant=w810:variant, value=w808:bool, error out=w809:errorcluster)  [unwired: 1 out]
            n156 = To Variant(anything=w808) -> (Variant=w806:variant)
          }
          frame True {
            n157 = Variant To Data(error in=w818, type=w819, Variant=w814) -> (data=w817:bool, error out=w816:errorcluster)
            n158 = Set Variant Attribute(Variant=w822, name=w821, value=w817, error in=w816) -> (Variant out=w820:variant, error out=w815:errorcluster)  [unwired: 1 out]
          }
        }
      }
      frame "UI Settings:Verbose Settings" {
        n159 = case shown="False" w831 {
          tunnel: w830 -> [w839 w848]
          tunnel: w829 -> [w838 w847]
          tunnel: [w836 w846] -> w828
          tunnel: "Verbose Settings" -> [w833 w845]
          tunnel: w827 -> [w837 w844]
          tunnel: w826 -> [_ w840]
          tunnel: [w835 w841] -> w825
          tunnel: [w832 w840] -> w824
          frame False {
            n160 = Get Variant Attribute(Variant=w839, name=w838, default value (empty Variant)=w833, error in=w837) -> (duplicate Variant=w836:variant, value=w834:bool, error out=w835:errorcluster)  [unwired: 1 out]
            n161 = To Variant(anything=w834) -> (Variant=w832:variant)
          }
          frame True {
            n162 = Variant To Data(error in=w844, type=w845, Variant=w840) -> (data=w843:bool, error out=w842:errorcluster)
            n163 = Set Variant Attribute(Variant=w848, name=w847, value=w843, error in=w842) -> (Variant out=w846:variant, error out=w841:errorcluster)  [unwired: 1 out]
          }
        }
      }
      frame "UI Settings:Verbose Saving" {
        n164 = case shown="False" w857 {
          tunnel: w856 -> [w865 w874]
          tunnel: w855 -> [w864 w873]
          tunnel: [w862 w872] -> w854
          tunnel: "Verbose Saving" -> [w859 w871]
          tunnel: w853 -> [w863 w870]
          tunnel: w852 -> [_ w866]
          tunnel: [w861 w867] -> w851
          tunnel: [w858 w866] -> w850
          frame False {
            n165 = Get Variant Attribute(Variant=w865, name=w864, default value (empty Variant)=w859, error in=w863) -> (duplicate Variant=w862:variant, value=w860:bool, error out=w861:errorcluster)  [unwired: 1 out]
            n166 = To Variant(anything=w860) -> (Variant=w858:variant)
          }
          frame True {
            n167 = Variant To Data(error in=w870, type=w871, Variant=w866) -> (data=w869:bool, error out=w868:errorcluster)
            n168 = Set Variant Attribute(Variant=w874, name=w873, value=w869, error in=w868) -> (Variant out=w872:variant, error out=w867:errorcluster)  [unwired: 1 out]
          }
        }
      }
    }
  }
  "Error Out" <- w2
  "Variant Data out" <- w1
